vi "Tbl_Delete (SubVI).vi"(11 "Table in":refnum<vi>) -> ()   [LabVIEW 2017]
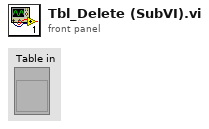
[diagram p1: front panel]
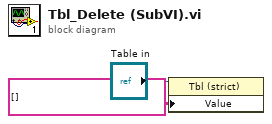
[diagram p0: block diagram]
diagram:
  n1 = property class="Tbl (strict)"(reference="Table in", "Value"=string[][] [] ("Protocol")) -> ()  [unwired: 1 in, 2 out]
